vi "Search for cmd line arg tokens.vi"(8 "error in (no error)":errorcluster, 10 "look for tokens":string[](array[string]), 11 "table":string[](array[string])) -> (0 "error out":errorcluster, 1 "[5]":bool, 2 "[4]":bool, 3 "Found token table":bool[](array[boolean]), 4 "[2]":bool, 5 "[3]":bool, 6 "[1]":bool, 7 "[0]":bool)   [LabVIEW 2024]
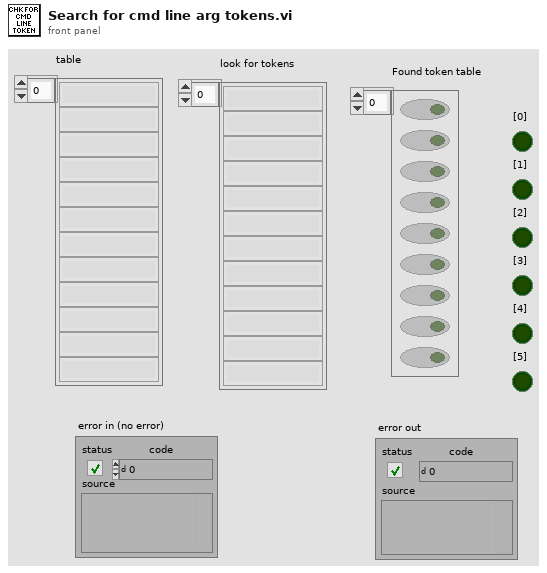
[diagram p1: front panel]
types:
  T1 = cluster{"[0]":bool, "[1]":bool, "[2]":bool, "[3]":bool, "[4]":bool, "[5]":bool, "[6]":bool, "[7]":bool, "[8]":bool}
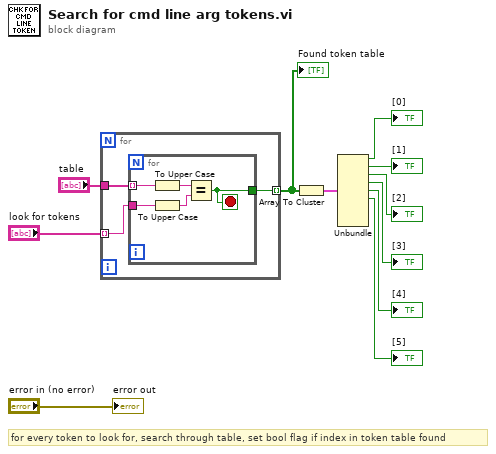
[diagram p0: block diagram]
diagram:
  # "for every token to look for, search through table, set bool flag if index in token table found"
  n1 = for {
    tunnel: "table" -> [w14]
    tunnel: "look for tokens" -> [w13] mode=indexing
    tunnel: [w12] -> w8 mode=indexing
    n2 = for {
      tunnel: w14 -> [w19] mode=indexing
      tunnel: w13 -> [w16]
      tunnel: [w18] -> w12
      stop <- w18 stop-if-true
      n3 = To Upper Case(1:w19) -> (0:w17:string)
      n4 = To Upper Case(1:w16) -> (0:w15:string)
      n5 = Equal?(x=w17, y=w15) -> (x = y?=w18:bool)
    }
  }
  "Found token table" <- w8
  n6 = Array To Cluster(array=w8) -> (cluster=w7:T1)
  n7 = Unbundle(w7) -> ("[0]"=→"[0]":bool, "[1]"=→"[1]":bool, "[2]"=→"[2]":bool, "[3]"=→"[3]":bool, "[4]"=→"[4]":bool, "[5]"=→"[5]":bool)  [unwired: 3 out]
  "error out" <- "error in (no error)"
